vi "solar_qtimer EnQ.vi"(8 "error in (no error)":errorcluster, 9 "Create if not found? (F)":bool, 10 "CMD (\"\")":string, 11 "QTimer Name":string) -> (0 "error out":errorcluster, 3 "QTimer":refnum<queue>, 5 "All QTimers":refnum<queue>[](array[refnum]))   [LabVIEW 2018]
doc: "[DEPRECIATED] This looks up and creates a new QTimer reference if it does not exist. All QTimers are maintained in this functional global."
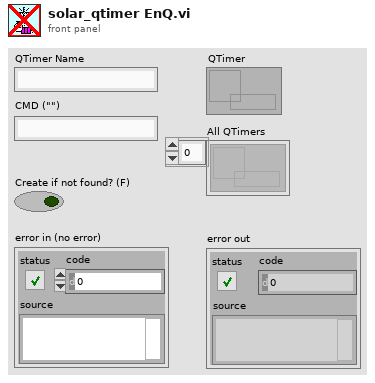
[diagram p1: front panel]
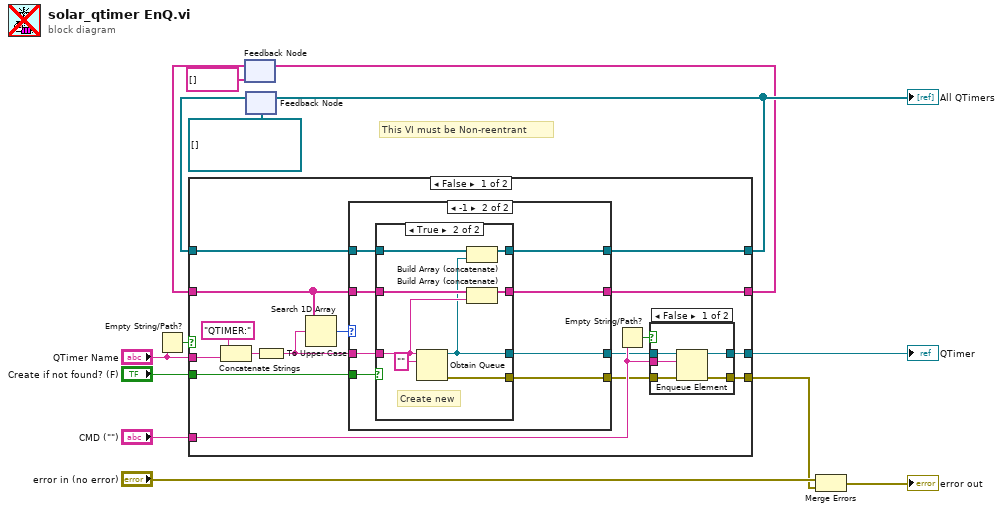
[diagram p0: block diagram]
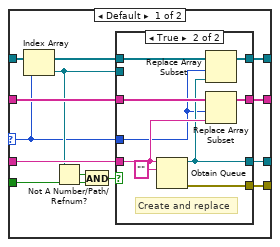
[diagram p2: hidden frame]
diagram:
  # "This VI must be Non-reentrant"
  n1 = Empty String/Path?(string/path="QTimer Name") -> (empty?=w2:bool)
  n2 = feedback #1(string[] []) -> (w6:string[])
  n3 = feedback #2(refnum<queue>[] [] ("queue out")) -> (w7:refnum<queue>[])
  n4 = case shown="False" w2 {
    tunnel: "QTimer Name" -> [w28 _]
    tunnel: [w27 _] -> w12
    tunnel: [w26 _] -> w11
    tunnel: "CMD (\"\")" -> [w25 _]
    tunnel: w7 -> [w21 w81]
    tunnel: w6 -> [w20 w80]
    tunnel: [w19 w81] -> w5
    tunnel: [w18 w80] -> w1
    tunnel: "Create if not found? (F)" -> [w16 _]
    frame False {
      n5 = Concatenate Strings("QTIMER:" ("string"), w28) -> (w30:string)
      n6 = To Upper Case(1:w30) -> (0:w23:string)
      n7 = Search 1D Array(1D array=w20, element=w23) -> (index of element=w22:i32)  [unwired: 1 in]
      n8 = case shown="-1" w22 {
        selector: w22 -> [w31 _]
        tunnel: w23 -> [w35 w57]
        tunnel: w21 -> [w39 w62]
        tunnel: [w38 w60] -> w19
        tunnel: [w37 w59] -> w18
        tunnel: w20 -> [w40 w61]
        tunnel: [w33 w56] -> w17
        tunnel: w16 -> [w41 w58]
        tunnel: [w32 w55] -> w15
        frame Default {
          n9 = Index Array(array=w39, index=w31) -> (element=w34:refnum<queue>)
          n10 = Not A Number/Path/Refnum?(number/path/refnum=w34) -> (NaN/Path/Refnum?=w42:bool)
          n11 = And(x=w42, y=w41) -> (x .and. y?=w36:bool)
          n12 = case shown="True" w36 {
            tunnel: [w45 w48] -> w38
            tunnel: w39 -> [w45 w49]
            tunnel: [w44 w51] -> w37
            tunnel: w40 -> [w44 w52]
            tunnel: [w43 w47] -> w33
            tunnel: w35 -> [_ w50]
            tunnel: [_ w53] -> w32
            tunnel: w34 -> [w43 _]
            tunnel: w31 -> [_ w46]
            frame False {
              # "Return existing"
            }
            frame True {
              # "Create and replace"
              n13 = Obtain Queue(name (unnamed)=w50, element data type="") -> (queue out=w47:refnum<queue>, error out=w53:errorcluster)  [unwired: 3 in, 1 out]
              n14 = Replace Array Subset(array=w49, new element=w47, index=w46) -> (w48:refnum<queue>[])
              n15 = Replace Array Subset(array=w52, new element=w50, index=w46) -> (w51:string[])
            }
          }
        }
        frame -1 {
          n16 = case shown="True" w58 {
            tunnel: [w64 w67] -> w60
            tunnel: w62 -> [w64 w71]
            tunnel: [w63 w69] -> w59
            tunnel: w61 -> [w63 w70]
            tunnel: [_ w66] -> w56
            tunnel: w57 -> [_ w68]
            tunnel: [_ w65] -> w55
            frame False {
              # "Do not create"
            }
            frame True {
              # "Create new"
              n17 = Obtain Queue(name (unnamed)=w68, element data type="") -> (queue out=w66:refnum<queue>, error out=w65:errorcluster)  [unwired: 3 in, 1 out]
              n18 = Build Array (concatenate)(w71, w66) -> (w67:refnum<queue>[])
              n19 = Build Array (concatenate)(w70, w68) -> (w69:string[])
            }
          }
        }
      }
      n20 = Empty String/Path?(string/path=w25) -> (empty?=w24:bool)
      n21 = case shown="False" w24 {
        tunnel: w17 -> [w77 w79]
        tunnel: [w76 w79] -> w27
        tunnel: w15 -> [w75 w78]
        tunnel: [w74 w78] -> w26
        tunnel: w25 -> [w73 _]
        frame False {
          n22 = Enqueue Element(queue=w77, element=w73, error in (no error)=w75) -> (queue out=w76:refnum<queue>, error out=w74:errorcluster)  [unwired: 1 in, 1 out]
        }
        frame True {
        }
      }
    }
    frame True {
    }
  }
  "QTimer" <- w12
  "All QTimers" <- w5
  n23 = feedback-in #1(w1) -> ()
  n24 = feedback-in #2(w5) -> ()
  n25 = Merge Errors("error in (no error)", w11) -> (→"error out":errorcluster)
